vi "estiUk.vi"(7 "Filter Type":T1, 8 "error in (no error)":errorcluster, 9 "Sensor Name":string[](array[string])=["R:4,4 S:0,0", "R:0,4 S:2,0", "R:0,0 S:2,2", "R:4,0 S:0,2"], 10 "Wavefront Error":dbl[][](array[numeric]), 11 "ZTAAC in":refnum<class "ZTAAC.lvclass">) -> (0 "error out":errorcluster, 2 "uk Array":dbl[](array[numeric]), 3 "ZTAAC out":refnum<class "ZTAAC.lvclass">)   [LabVIEW 2016, in "ZTAAC.lvclass"]
doc: "Estimate uk by referencing to \"0\", \"x0\", or \"x00\" based on the configuration file. The inputs are the filter type, wavefront error, and sensor name list."
uses:
  ZTAAC.lvclass
  StrictDef/FilterType.ctl
  ZTAAC.lvclass/ZTAAC.ctl
  OptStateEsti/OptStateEsti.lvclass
  OptCtrl/OptCtrl.lvclass
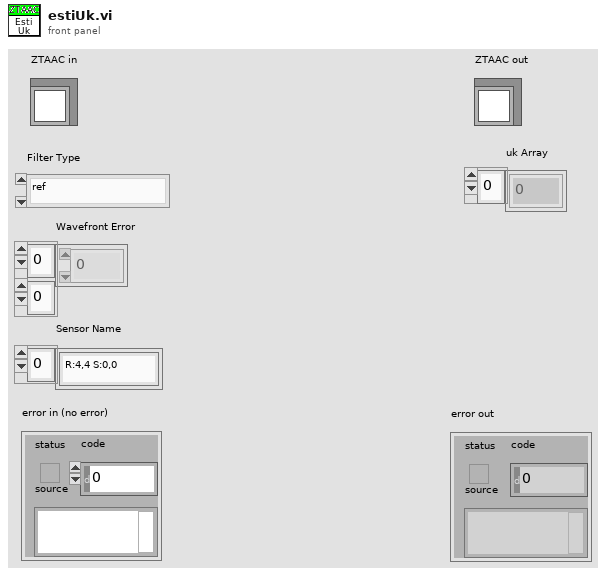
[diagram p1: front panel]
types:
  T1 = typedef "FilterType.ctl" = enum16{"ref", "u", "g", "r", "i", "z", "y"}
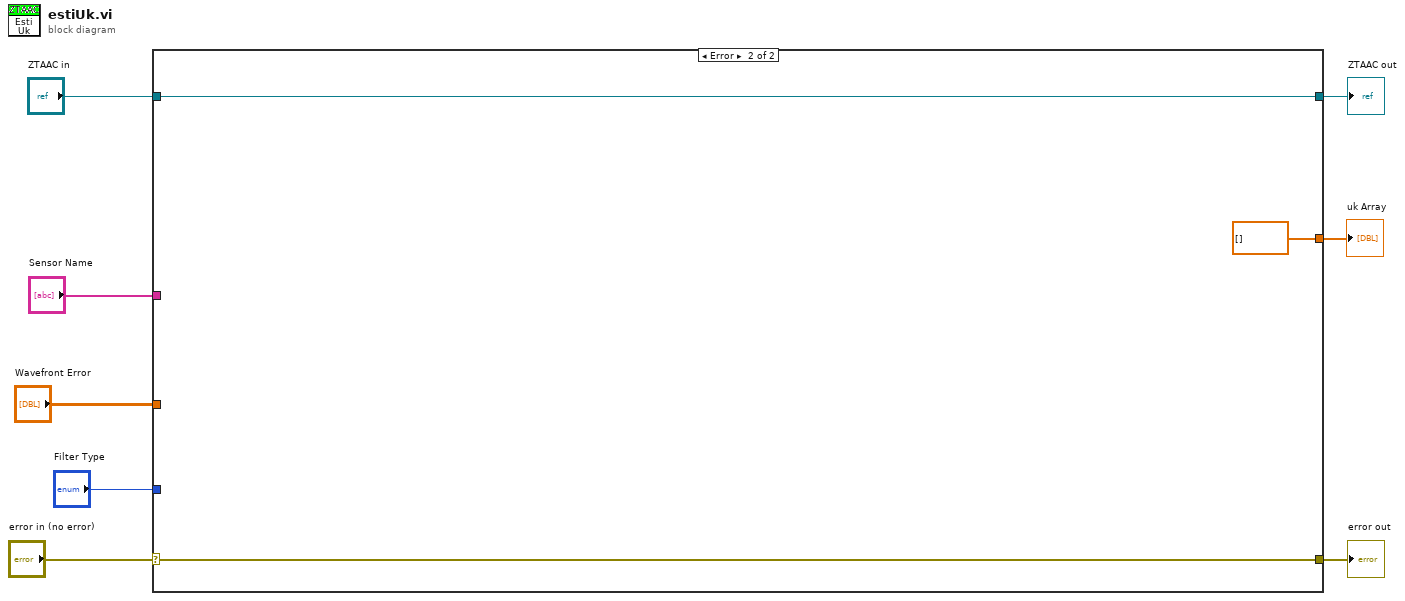
[diagram p0: block diagram]
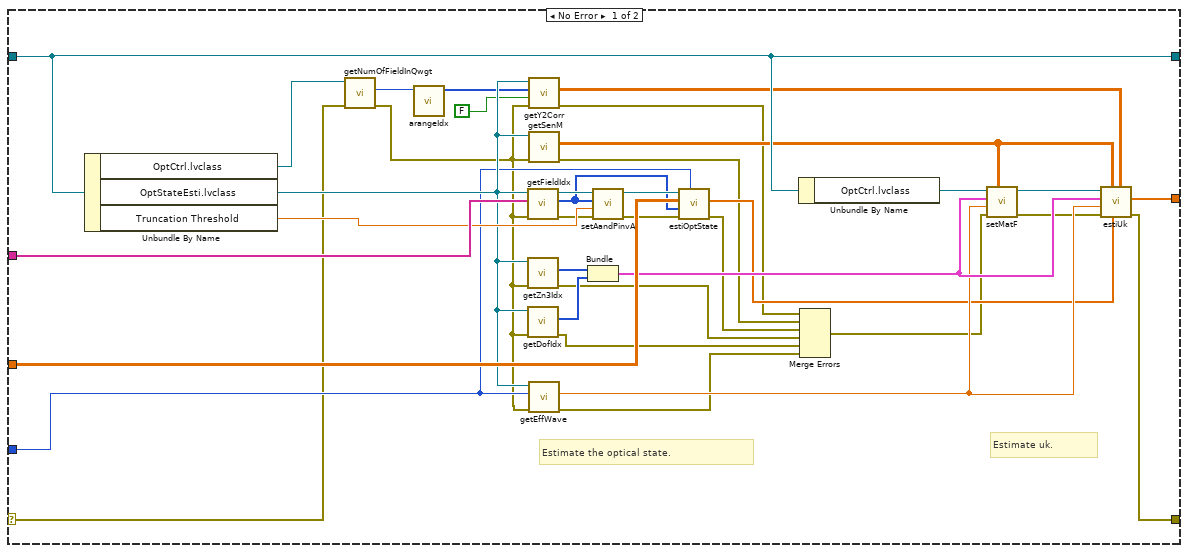
[diagram p2: hidden frame]
diagram:
  n1 = case shown="Error" "error in (no error)" {
    selector: "error in (no error)" -> [w10 w47]
    tunnel: [w13 w47] -> w7
    tunnel: [w39 w46] -> w5
    tunnel: "ZTAAC in" -> [w39 w46]
    tunnel: "Sensor Name" -> [w44 _]
    tunnel: "Wavefront Error" -> [w41 _]
    tunnel: "Filter Type" -> [w20 _]
    tunnel: [w27 dbl[] [] ("uk Array")] -> w1
    frame No Error {
      # "Estimate uk."
      # "Estimate the optical state."
      n2 = Unbundle By Name(w39) -> ("OptCtrl.lvclass"=w12:refnum<class "OptCtrl.lvclass">, "OptStateEsti.lvclass"=w31:refnum<class "OptStateEsti.lvclass">, "Truncation Threshold"=w38:dbl)
      n3 = call "getNumOfFieldInQwgt.vi"("error in (no error)"=w10, "OptCtrl in"=w12) -> ("error out"=w9:errorcluster, "Num of Field"=w11:i32)  [unwired: 7 in, 1 out]
      n4 = call "arangeIdx.vi"("Number"=w11) -> ("Idx Array"=w30:i32[])  [unwired: 10 in]
      n5 = call "getFieldIdx.vi"("error in (no error)"=w9, "Sensor Name"=w44, "OptStateEsti in"=w31) -> ("error out"=w24:errorcluster, "Field Idx"=w40:i32[], "OptStateEsti out"=w43:refnum<class "OptStateEsti.lvclass">)  [unwired: 6 in]
      n6 = call "getZn3Idx.vi"("error in (no error)"=w9, "OptStateEsti in"=w31) -> ("error out"=w18:errorcluster, "zn3Idx"=w37:i32[])  [unwired: 7 in, 1 out]
      n7 = call "getDofIdx.vi"("error in (no error)"=w9, "OptStateEsti in"=w31) -> ("error out"=w17:errorcluster, "dofIdx"=w36:i32[])  [unwired: 7 in, 1 out]
      n8 = call "getY2Corr.vi"("error in (no error)"=w9, "In nx1 Row"=FALSE, "Field Idx"=w30, "OptStateEsti in"=w31) -> ("error out"=w22:errorcluster, "y2c Array"=w28:dbl[][])  [unwired: 5 in, 1 out]
      n9 = call "getSenM.vi"("error in (no error)"=w9, "OptStateEsti in"=w31) -> ("error out"=w21:errorcluster, "Sen M"=w25:dbl[][][])  [unwired: 7 in, 1 out]
      n10 = call "getEffWave.vi"("error in (no error)"=w9, "Filter Type"=w20, "OptStateEsti in"=w31) -> ("error out"=w16:errorcluster, "Effective Wavelength  (um)"=w33:dbl)  [unwired: 6 in, 1 out]
      n11 = Bundle("zn3Idx"=w37, "dofIdx"=w36) -> (w34:cluster{"zn3Idx":i32[], "dofIdx":i32[]})  [unwired: 1 in]
      n12 = call "setAandPinvA.vi"("error in (no error)"=w24, "Truncation Threshold"=w38, "Field Idx"=w40, "OptStateEsti in"=w43) -> ("error out"=w23:errorcluster, "OptStateEsti out"=w42:refnum<class "OptStateEsti.lvclass">)  [unwired: 6 in]
      n13 = call "estiOptState.vi"("Filter Type"=w20, "error in (no error)"=w23, "Field Idx"=w40, "Zk"=w41, "OptStateEsti in"=w42) -> ("error out"=w19:errorcluster, "Optical State"=w32:dbl[])  [unwired: 4 in, 1 out]
      n14 = Unbundle By Name(w39) -> ("OptCtrl.lvclass"=w26:refnum<class "OptCtrl.lvclass">)
      n15 = Merge Errors(w22, w21, w19, w18, w17, w16) -> (w15:errorcluster)
      n16 = call "setMatF.vi"("Sen M"=w25, "error in (no error)"=w15, "Effective Wavelength"=w33, "Idx Group"=w34, "OptCtrl in"=w26) -> ("error out"=w14:errorcluster, "OptCtrl out"=w35:refnum<class "OptCtrl.lvclass">)  [unwired: 5 in]
      n17 = call "estiUk.vi"("y2 Matrix"=w28, "Optical State"=w32, "Sen M"=w25, "error in (no error)"=w14, "Effective Wavelength"=w33, "Idx Group"=w34, "OptCtrl in"=w35) -> ("error out"=w13:errorcluster, "uk Array"=w27:dbl[])  [unwired: 2 in, 1 out]
    }
    frame Error {
    }
  }
  "error out" <- w7
  "ZTAAC out" <- w5
  "uk Array" <- w1
